vi "Append Image to Report.vi"(5 "alignment (default)":T2, 6 "error in (no error)":errorcluster, 7 "caption or alternative string":string, 8 "path or URL of image":string, 9 "report in":T1) -> (0 "error out":errorcluster, 3 "report out":T1)   [LabVIEW 2017]
doc: "For an HTML report, the VI embeds a link to an image into the report. For a standard report, the VI appends the image from a file."
uses:
  <vilib>/Utility/NIReport.llb/HTML Report Image Alignment.ctl
  <vilib>/Utility/NIReport.llb/Generate Report Object Reference.ctl
  <vilib>/Utility/NIReport.llb/NI_report.lvclass
  <vilib>/Utility/NIReport.llb/NI_ReportGenerationCore.lvlib
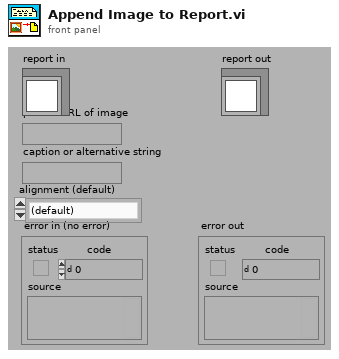
[diagram p1: front panel]
types:
  T1 = typedef "Generate Report Object Reference.ctl" = refnum<class "NI_report.lvclass">
  T2 = typedef "NI_ReportGenerationCore.lvlib/HTML Report Image Alignment.ctl" = enum16{"(default)", "LEFT", "RIGHT", "TOP", "TEXTTOP", "MIDDLE", "ABSMIDDLE", "BASELINE", "BOTTOM", "ABSBOTTOM"}
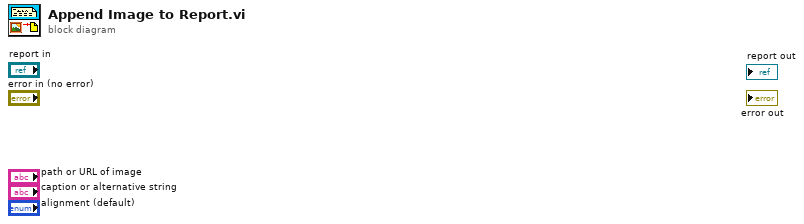
[diagram p0: block diagram]
diagram:
